vi "Is Within Time Threshold.vi"(6 "error in (no error)":errorcluster, 8 "Time gauge [ms]":dbl(knob)=150.0 scale=0.0..1000.0, 9 "Current Cluster Array":T1(array[cluster]), 10 "Input array":dbl[](array[numeric])) -> (1 "Threshold?":bool, 4 "error IO":errorcluster)   [LabVIEW 2014]
doc: "This VI checks wether given input with a time variable is within the supplied time threshold. The input is given by an input file which is read in by the 'Read In' VI to cluster each data entry (row) appriopiately according to the time threshold."
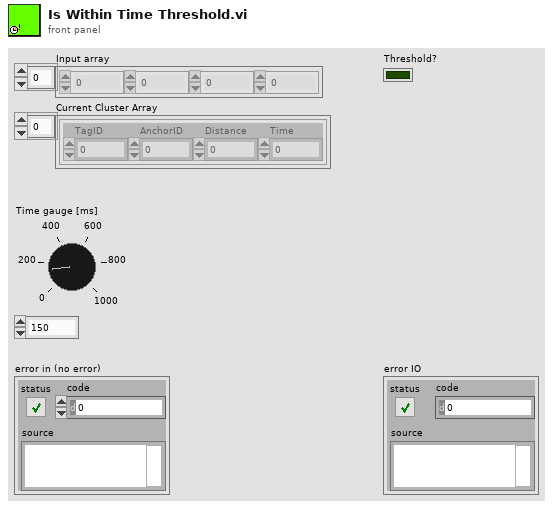
[diagram p1: front panel]
types:
  T1 = cluster{"TagID":dbl, "AnchorID":dbl, "Distance":dbl, "Time":dbl}[]
  T2 = cluster{"TagID":dbl, "AnchorID":dbl, "Distance":dbl, "Time":dbl}
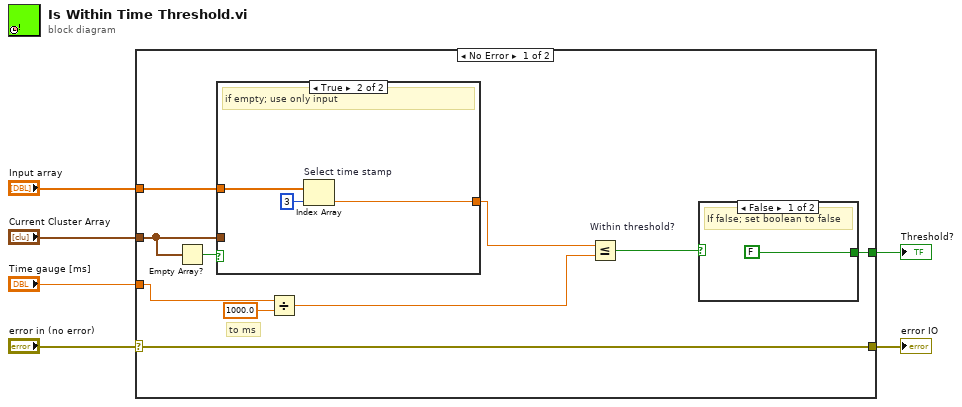
[diagram p0: block diagram]
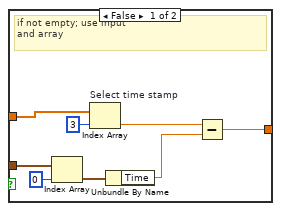
[diagram p2: hidden frame]
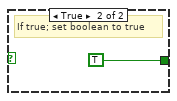
[diagram p3: hidden frame]
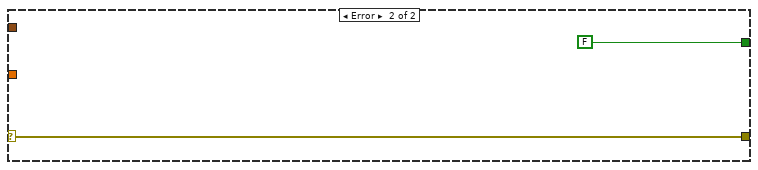
[diagram p4: hidden frame]
diagram:
  n1 = case shown="No Error" "error in (no error)" {
    selector: "error in (no error)" -> [w14 w31]
    tunnel: "Input array" -> [w11 _]
    tunnel: [w15 FALSE] -> w5
    tunnel: "Current Cluster Array" -> [w12 _]
    tunnel: "Time gauge [ms]" -> [w9 _]
    tunnel: [w14 w31] -> w1
    frame No Error {
      # "to ms"
      n2 = Empty Array?(array=w12) -> (empty?=w13:bool)
      n3 = case shown="True" w13 {
        tunnel: w12 -> [w22 _]
        tunnel: [w20 w25] -> w10
        tunnel: w11 -> [w18 w26]
        frame False {
          # "if not empty; use input \nand array"
          n4 = Index Array "Index Array"(array=w22, index=0) -> (element=w23:T2)
          n5 = Index Array "Select time stamp"(array=w18, index=3) -> (element=w17:dbl)
          n6 = Unbundle By Name(w23) -> ("Time"=w21:dbl)
          n7 = Subtract(x=w17, y=w21) -> (x-y=w20:dbl)
        }
        frame True {
          # "if empty; use only input"
          n8 = Index Array "Select time stamp"(array=w26, index=3) -> (element=w25:dbl)
        }
      }
      n9 = Divide(x=w9, y=1000.0) -> (x/y=w7:dbl)
      n10 = Less Or Equal? "Within threshold?"(x=w10, y=w7) -> (x <= y?=w16:bool)
      n11 = case shown="False" w16 {
        tunnel: [FALSE TRUE] -> w15
        frame False {
          # "If false; set boolean to false"
        }
        frame True {
          # "If true; set boolean to true"
        }
      }
    }
    frame Error {
    }
  }
  "Threshold?" <- w5
  "error IO" <- w1
